vi "Experiment header-Write keys.vi"(8 "error in (no error)":errorcluster, 10 "Section Refs":T2[](array[typedef]), 11 "FIle refnum IN":T1) -> (0 "error in (no error) 2":errorcluster, 3 "FIle refnum OUT":T1)   [LabVIEW 2017]
uses:
  Typedefs/Header file section refs.ctl
  <vilib>/Utility/config.llb/Config Data RefNum.ctl
  <vilib>/Utility/Data Type/NI_Data Type.lvlib
  <vilib>/Utility/config.llb/NI_LVConfig.lvlib
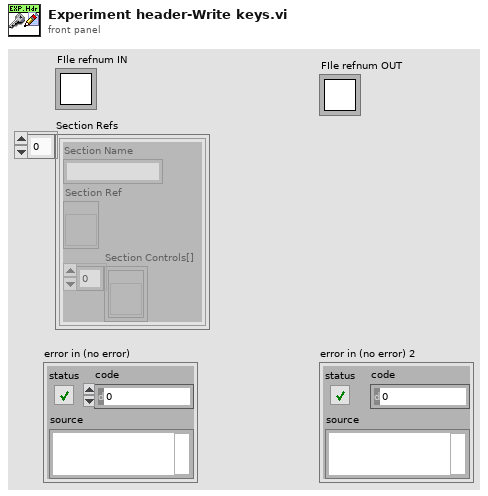
[diagram p1: front panel]
types:
  T1 = typedef "NI_LVConfig.lvlib/Config Data RefNum.ctl" = refnum<k1>
  T2 = typedef "Header file section refs.ctl" = cluster{"Section Name":string, "Section Ref":refnum<vi>, "Section Controls[]":refnum<vi>[]}
  T3 = typedef "NI_Data Type.lvlib/Data Type.ctl" = enum8{"Invalid Type", "Void", "I8", "I16", "I32", "I64", "U8", "U16", "U32", "U64", "Single Float", "Double Float", "Extended Float", "Single Complex", "Double Complex", "Extended Complex", "Enum U8", "Enum U16", "Enum U32", "Enum U64", "Single Float With Unit", "Double Float With Unit", "Extended Float With Unit", "Single Complex with Unit", "Double Complex with Unit", "Extended Complex with Unit", "Boolean", "String", "Path", "Picture", "Tag", "Array", "Cluster", "Variant", "LV Variant", "Waveform", "Timestamp", "Digital Waveform", "Digital Data", "ExpressData", "Refnum", "External Data", "VI", "Poly VI", "LabVIEW Class Instance", "Fixed Point"}
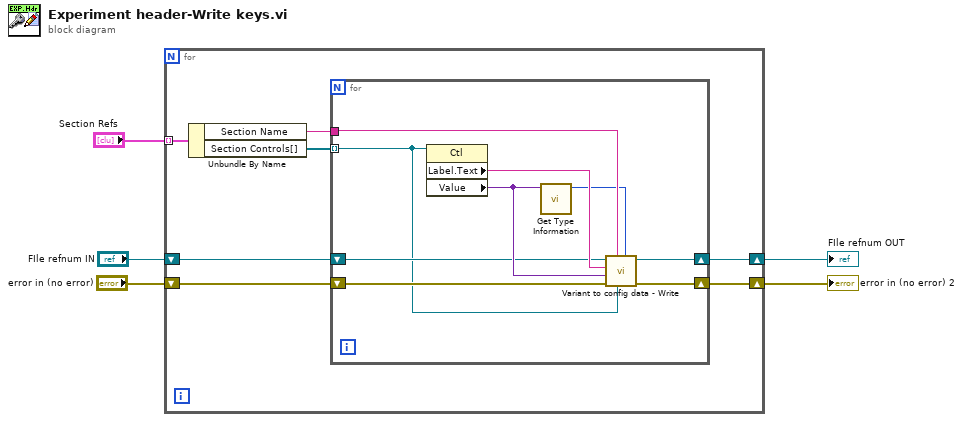
[diagram p0: block diagram]
diagram:
  n1 = for {
    tunnel: "Section Refs" -> [w12] mode=indexing
    shift-right: [w8] -> w2
    shift-left: "FIle refnum IN" -> [w9]
    shift-right: [w6] -> w1
    shift-left: "error in (no error)" -> [w7]
    n2 = Unbundle By Name(w12) -> ("Section Name"=w11:string, "Section Controls[]"=w10:refnum<vi>[])
    n3 = for {
      tunnel: w11 -> [w21]
      tunnel: w10 -> [w13] mode=indexing
      shift-right: [w16] -> w8
      shift-left: w9 -> [w17]
      shift-right: [w14] -> w6
      shift-left: w7 -> [w15]
      n4 = property class="Ctl"(reference=w13) -> ("Label.Text"=w20:string, "Value"=w18:variant)  [unwired: 1 in, 2 out]
      n5 = call <vilib>:"Get Type Information.vi"("Variant"=w18) -> ("Type"=w19:T3)  [unwired: 6 in, 4 out]
      n6 = call "Variant to config data - Write.vi"("Type"=w19, "Control in"=w13, "Section Name"=w21, "error in (no error)"=w15, "Value"=w18, "Key Name"=w20, "FIle refnum IN"=w17) -> ("error out"=w14:errorcluster, "Refnum out"=w16:T1)  [unwired: 3 in]
    }
  }
  "FIle refnum OUT" <- w2
  "error in (no error) 2" <- w1
